vi "long_grid.vi"(0 "pict in":picture, 1 "size":i32=40, 2 "nr lines":cluster{"x":i32, "y":i32}={"x"=7, "y"=15}, 3 "rotation":dbl[][](array[numeric]), 4 "Half sphere":bool, 5 "center":cluster{"x":i32, "y":i32}={"x"=44, "y"=44}) -> (6 "pict out":picture)   [LabVIEW 2011]
uses:
  <vilib>/Analysis/baseanly.llb/Real A x B.vi
  <vilib>/Analysis/NI_AALBase.lvlib
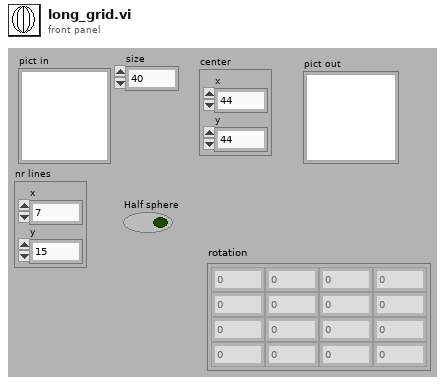
[diagram p1: front panel]
types:
  T1 = typedef "NI_Matrix.lvlib/RealMatrix.ctl" = dbl[][]
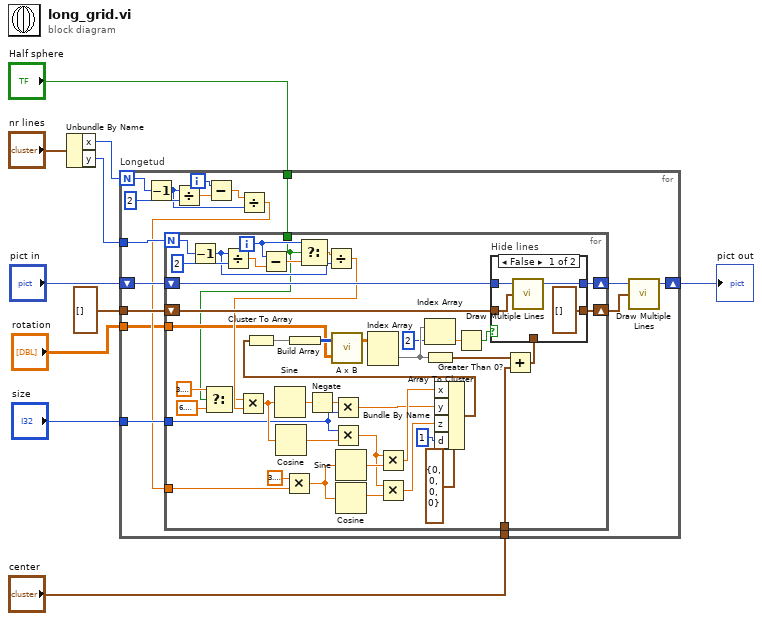
[diagram p0: block diagram]
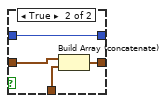
[diagram p2: hidden frame]
diagram:
  n1 = Unbundle By Name("nr lines") -> ("x"=w7:i32, "y"=w8:i32)
  n2 = for "Longetud" {
    N: w7 -> [w24]
    tunnel: w8 -> [w27]
    shift-right: [w20] -> w3
    shift-left: "pict in" -> [w22]
    tunnel: "size" -> [w23]
    tunnel: cluster{"A x B[0]":dbl, "A x B[1]":dbl}[] [] -> [w18]
    tunnel: "rotation" -> [w15]
    tunnel: "center" -> [w14]
    tunnel: "Half sphere" -> [w11]
    i -> [w13]
    n3 = Decrement(x=w24) -> (x-1=w17:i32)
    n4 = Divide(x=w17, y=2) -> (x/y=w25:dbl)
    n5 = Subtract(x=w13, y=w25) -> (x-y=w12:dbl)
    n6 = Divide(x=w12, y=w17) -> (x/y=w16:dbl)
    n7 = for {
      N: w27 -> [w66]
      tunnel: w23 -> [w39]
      shift-right: [w64] -> w19
      shift-left: w18 -> [w63]
      shift-right: [w57] -> w21
      shift-left: w22 -> [w58]
      tunnel: w16 -> [w53]
      tunnel: w15 -> [w50]
      tunnel: w14 -> [w37]
      tunnel: w11 -> [w28]
      i -> [w34]
      n8 = Decrement(x=w66) -> (x-1=w65:i32)
      n9 = Select(t=3.141592653589793, s=w28, f=6.283185307179586) -> (s? t:f=w32:dbl)
      n10 = Divide(x=w65, y=2) -> (x/y=w68:dbl)
      n11 = Subtract(x=w34, y=w68) -> (x-y=w35:dbl)
      n12 = Multiply(x=3.141592653589793, y=w53) -> (x*y=w48:dbl)
      n13 = Select(t=w34, s=w28, f=w35) -> (s? t:f=w33:dbl)
      n14 = Divide(x=w33, y=w65) -> (x/y=w54:dbl)
      n15 = Multiply(x=w32, y=w54) -> (x*y=w44:dbl)
      n16 = Sine(x=w44) -> (sin(x)=w49:dbl)
      n17 = Cosine(x=w44) -> (cos(x)=w40:dbl)
      n18 = Negate(x=w49) -> (-x=w36:dbl)
      n19 = Multiply(x=w36, y=w39) -> (x*y=w41:dbl)
      n20 = Multiply(x=w39, y=w40) -> (x*y=w43:dbl)
      n21 = Sine(x=w48) -> (sin(x)=w47:dbl)
      n22 = Cosine(x=w48) -> (cos(x)=w46:dbl)
      n23 = Multiply(x=w43, y=w47) -> (x*y=w45:dbl)
      n24 = Multiply(x=w43, y=w46) -> (x*y=w42:dbl)
      n25 = Bundle By Name(cluster=cluster{"x":i16, "y":i16, "z":i16, "d":i16} {"x"=0, "y"=0, "z"=0, "d"=0}, "x"=w45, "y"=w41, "z"=w42, "d"=i16 1) -> (w71:cluster{"x":i16, "y":i16, "z":i16, "d":i16})
      n26 = Cluster To Array(cluster=w71) -> (array=w70:i16[])
      n27 = Build Array(w70) -> (w52:i16[][])
      n28 = call-poly <vilib>:"A x B.vi"("B"=w50, "A"=w52) -> ("A x B"=w51:T1)  [unwired: 1 out]
      n29 = Index Array(array=w51) -> (element=w62:dbl[])  [unwired: 2 in]
      n30 = Index Array(array=w62, index=2) -> (element=w61:dbl)
      n31 = Array To Cluster(array=w62) -> (cluster=w56:cluster{"A x B[0]":dbl, "A x B[1]":dbl})
      n32 = Greater Than 0?(x=w61) -> (x > 0?=w60:bool)
      n33 = Add(x=w56, y=w37) -> (x+y=w55:cluster{dbl, dbl})
      n34 = case "Hide lines" shown="False" w60 {
        tunnel: [cluster{"A x B[0]":dbl, "A x B[1]":dbl}[] [] w79] -> w64
        tunnel: w63 -> [w72 w78]
        tunnel: w58 -> [w74 w77]
        tunnel: [w73 w77] -> w57
        tunnel: w55 -> [_ w76]
        frame False {
          n35 = call <vilib>:"Draw Multiple Lines.vi"("picture"=w74, "line endpoints"=w72) -> ("new picture"=w73:picture)  [unwired: 7 in]
        }
        frame True {
          n36 = Build Array (concatenate)(w78, w76) -> (w79:cluster{"A x B[0]":dbl, "A x B[1]":dbl}[])
        }
      }
    }
    n37 = call <vilib>:"Draw Multiple Lines.vi"("picture"=w21, "line endpoints"=w19) -> ("new picture"=w20:picture)  [unwired: 7 in]
  }
  "pict out" <- w3
